vi "UHR-Fleezers Control (host) - 11.1.vi"() -> ()   [LabVIEW 2012] (continued)
        n1599 = feedback #34() -> (w2754:u32)  [unwired: 1 out]
        n1600 = case shown="True" w2761 {
          tunnel: [w2773 1] -> w2762
          tunnel: w2766 -> [w2775 _]
          tunnel: [w2774 w2793] -> w2763
          tunnel: w2764 -> [w2774 _]
          tunnel: w2760 -> [_ w2813]
          tunnel: w2753 -> [_ w2811]
          tunnel: w2755 -> [_ w2814]
          tunnel: [w2772 w2792] -> w2752
          tunnel: w2754 -> [w2772 _]
          tunnel: [w2771 w2790] -> w2749
          tunnel: w2750 -> [w2771 _]
          tunnel: [w2770 w2789] -> w2746
          tunnel: w2747 -> [w2770 _]
          tunnel: "Start Saving" -> [_ w2787]
          tunnel: w2742 -> [_ w2786]
          tunnel: [w2769 w2777] -> w2735
          tunnel: w2739 -> [w2769 _]
          tunnel: [w2768 w2776] -> w2736
          tunnel: w2737 -> [w2768 _]
          frame False {
            n1601 = Increment(x=w2775) -> (x+1=w2773:i32)
          }
          frame True {
            w2783 = FALSE ("Start Saving")
            w2788 = 9.0  # File Version
            w2796 = FALSE ("prepend array or string size? (T)")
            w2794 = T36."big-endian, network order" ("byte order (0:big-endian, network order)")
            n1602 = local read "BD 1 Frequency 1 (MHz)"() -> (w2810:dbl)
            n1603 = local read "BD 2 Frequency 1 (MHz)"() -> (w2809:dbl)
            n1604 = local read "BD 1 Frequency 2 (MHz)"() -> (w2808:dbl)
            n1605 = local read "BD 2 Frequency 2 (MHz)"() -> (w2807:dbl)
            n1606 = local read "BD 1 Frequency 3 (MHz)"() -> (w2806:dbl)
            n1607 = local read "BD 2 Frequency 3 (MHz)"() -> (w2805:dbl)
            n1608 = Array Size(array=w2786) -> (size(s)=w2785:i32)
            n1609 = To Double Precision Float(number=w2785) -> (double precision float=w2784:dbl)
            n1610 = local write "Save Calibration"(w2783) -> ()
            n1611 = local write "Start Saving"(w2783) -> ()
            n1612 = Build Array("Save APD Data\nwith Trap Data", "Save Trap Pos. Data") -> (w2780:bool[])
            n1613 = Boolean Array To Number(Boolean array=w2780) -> (number=w2779:u32)
            n1614 = Build Array(w2810, w2809, w2808, w2807, w2806, w2805) -> (w2804:dbl[])
            n1615 = case shown="1, Default" w2814 {
              tunnel: w2813 -> [w2885 w2905 w2921 w2959]
              tunnel: w2784 -> [w2890 w2912 w2941 w2978]
              tunnel: w2811 -> [w2889 w2911 w2940 w2977]
              tunnel: [w2886 w2907 w2932 w2969] -> w2802
              tunnel: [w2877 "Cal sets to save" w2922 w2960] -> w2792
              tunnel: w2804 -> [w2887 w2908 w2934 w2971]
              tunnel: "Save APD Data\nwith Trap Data" -> [w2884 _ w2918 w2957]
              tunnel: [w2884 w2899 w2918 w2957] -> w2789
              tunnel: w2788 -> [w2880 w2900 w2916 w2955]
              tunnel: w2787 -> [w2879 _ _ _]
              tunnel: [w2870 w2899 w2915 w2945] -> w2776
              tunnel: "Save Trap Pos. Data" -> [w2870 _ w2915 w2945]
              tunnel: w2779 -> [w2869 _ w2914 w2944]
              frame 1, Default {
                # "timeseries"
                n1616 = case shown="True" "Profile" {
                  tunnel: [w2893 w2897] -> w2874
                  tunnel: [w2893 w2896] -> w2873
                  tunnel: [w2893 w2895] -> w2872
                  tunnel: [w2893 w2894] -> w2871
                  frame False {
                    w2893 = 0.0 ("f")
                  }
                  frame True {
                    n1617 = local read "Current Position"() -> (w2898:cluster{dbl, dbl, dbl})
                    n1618 = local read "Y change (mm)"() -> (w2894:dbl)
                    n1619 = Unbundle(w2898) -> (w2897:dbl, w2896:dbl, w2895:dbl)
                  }
                }
                n1620 = local read "Save ave N"() -> (w2892:dbl)
                n1621 = Multiply(x=w2892, y=w2885) -> (x*y=w2891:dbl)
                n1622 = To Double Precision Float(number=w2869) -> (double precision float=w2883:dbl)
                n1623 = Build Array(w2880, w2885, w2891, w2890, w2889, 0.0 ("f")) -> (w2888:dbl[])
                n1624 = Build Array(w2883, w2874, w2873, w2872, w2871) -> (w2881:dbl[])
                n1625 = Select(t=u32 4000000000, s=w2879, f="N sets to save") -> (s? t:f=w2877:u32)
                n1626 = Build Array (concatenate)(w2888, w2887, w2881) -> (w2886:dbl[])
              }
              frame 2 {
                w2902 = 0.0 ("f")
                w2899 = FALSE ("Save APD Data\nwith Trap Data")
                # "calibration"
                n1627 = Boolean To (0,1)(Boolean=w2899) -> (0, 1=w2904:i16)
                n1628 = To Double Precision Float(number=w2904) -> (double precision float=w2903:dbl)
                n1629 = Build Array(w2903, w2902, w2902, w2902, w2902) -> (w2901:dbl[])
                n1630 = Build Array(w2900, w2905, w2905, w2912, w2911, 1.0 ("t")) -> (w2909:dbl[])
                n1631 = Build Array (concatenate)(w2909, w2908, w2901) -> (w2907:dbl[])
                "Calibrating Trap..." <- TRUE ("Calibrating...")
              }
              frame 4 {
                w2919 = 0.0 ("f")
                # "scan dir (x/y = 0/1)"
                # "cycles/step"
                # "n scans (f/b)"
                # "steps"
                # "freq. range"
                # "AOD raster scan"
                n1632 = local read "Number of F/B Scans (AOD)"() -> (w2926:u16)
                n1633 = local read "Cycles/step (AOD)"() -> (w2928:u64)
                n1634 = local read "Scan Range (MHz)"() -> (w2931:dbl)
                n1635 = local read "Scan steps (AOD)"() -> (w2930:u64)
                n1636 = local read "Scan BD"() -> (w2938:bool)
                n1637 = local read "Save ave N"() -> (w2943:dbl)
                n1638 = Boolean To (0,1)(Boolean=w2938) -> (0, 1=w2937:i16)
                n1639 = To Double Precision Float(number=w2926) -> (double precision float=w2925:dbl)
                n1640 = To Double Precision Float(number=w2930) -> (double precision float=w2929:dbl)
                n1641 = To Double Precision Float(number=w2928) -> (double precision float=w2927:dbl)
                n1642 = To Double Precision Float(number=w2937) -> (double precision float=w2936:dbl)
                n1643 = Multiply(x=w2943, y=w2921) -> (x*y=w2942:dbl)
                n1644 = To Double Precision Float(number=w2914) -> (double precision float=w2920:dbl)
                n1645 = Build Array(w2920, w2919, w2919, w2919, w2919) -> (w2917:dbl[])
                n1646 = local read "N sets should be saved"() -> (w2923:dbl)
                n1647 = Build Array(w2936, w2931, w2929, w2927, w2925) -> (w2933:dbl[])
                n1648 = Build Array(w2916, w2921, w2942, w2941, w2940, 2.0 ("t")) -> (w2935:dbl[])
                n1649 = Round Toward +Infinity(x=w2923) -> (ceil(x): smallest int >= x=w2924:dbl)
                n1650 = Build Array (concatenate)(w2935, w2934, w2917, w2933) -> (w2932:dbl[])
                n1651 = To Unsigned Long Integer(number=w2924) -> (unsigned 32bit integer=w2922:u32)
              }
              frame 8 {
                w2952 = 0.0 ("f")
                # "MCL raster scan"
                n1652 = local read "Number of scans (MCL)"() -> (w2947:u64)
                n1653 = local read "Scan lines (y)"() -> (w2946:u64)
                n1654 = local read "2D or 1D Scan"() -> (w2949:bool)
                n1655 = local read "Scan Range (V)\n(of steps)"() -> (w2968:dbl)
                n1656 = local read "Fast Scan Dir"() -> (w2975:bool)
                n1657 = local read "Cycles/step (MCL)"() -> (w2965:u64)
                n1658 = local read "Scan steps (MCL)"() -> (w2967:u64)
                n1659 = Select(t=w2946, s=w2949, f=w2947) -> (s? t:f=w2948:u64)
                n1660 = Boolean To (0,1)(Boolean=w2949) -> (0, 1=w2951:i16)
                n1661 = local read "Save ave N"() -> (w2980:dbl)
                n1662 = local read "Initial X"() -> (w2954:dbl)
                n1663 = local read "Initial Y"() -> (w2953:dbl)
                n1664 = To Double Precision Float(number=w2951) -> (double precision float=w2950:dbl)
                n1665 = Boolean To (0,1)(Boolean=w2975) -> (0, 1=w2974:i16)
                n1666 = To Double Precision Float(number=w2948) -> (double precision float=w2963:dbl)
                n1667 = To Double Precision Float(number=w2967) -> (double precision float=w2966:dbl)
                n1668 = To Double Precision Float(number=w2965) -> (double precision float=w2964:dbl)
                n1669 = To Double Precision Float(number=w2974) -> (double precision float=w2973:dbl)
                n1670 = Multiply(x=w2980, y=w2959) -> (x*y=w2979:dbl)
                n1671 = To Double Precision Float(number=w2944) -> (double precision float=w2958:dbl)
                n1672 = local read "N sets should be saved (MCL)"() -> (w2961:dbl)
                n1673 = Build Array(w2958, w2950, w2952, w2952, w2952) -> (w2956:dbl[])
                n1674 = Build Array(w2973, w2968, w2966, w2964, w2963, w2954, w2953) -> (w2970:dbl[])
                n1675 = Build Array(w2955, w2959, w2979, w2978, w2977, 3.0 ("t")) -> (w2972:dbl[])
                n1676 = Round Toward +Infinity(x=w2961) -> (ceil(x): smallest int >= x=w2962:dbl)
                n1677 = Build Array (concatenate)(w2972, w2971, w2956, w2970) -> (w2969:dbl[])
                n1678 = To Unsigned Long Integer(number=w2962) -> (unsigned 32bit integer=w2960:u32)
              }
            }
            n1679 = local read "Index"() -> (w2819:dbl)
            n1680 = call "Create new save file.vi"("Insert"="", "Ext"=".dat", "Index In"=w2819) -> ("Path Out"=w2778:path, "Index Out"=w2791:dbl)
            n1681 = local write "Save file name"(w2778) -> ()
            n1682 = local write "Index"(w2791) -> ()
            n1683 = local write "Save index"(w2791) -> ()
            n1684 = Array Size(array=w2802) -> (size(s)=w2803:i32)
            n1685 = Open/Create/Replace File(file path (use dialog)=w2778, operation (0:open)=T35."create", access (0:read/write)=enum16{"read/write", "read-only", "write-only"}."write-only") -> (refnum out=w2816:refnum<file>)  [unwired: 1 in, 4 out]
            n1686 = local write "Saving..."(TRUE ("Saving...")) -> ()
            n1687 = To Double Precision Float(number=w2803) -> (double precision float=w2801:dbl)
            n1688 = String Length(string="Comment (data description)") -> (length=w2799:i32)
            n1689 = To Double Precision Float(number=w2799) -> (double precision float=w2798:dbl)
            n1690 = Deny Access(7:w2816) -> (3:w2815:refnum<file>)  [unwired: 1 in, 2 out]
            n1691 = Build Array (concatenate)(w2801, w2802, w2798) -> (w2800:dbl[])
            n1692 = case "If fluorescence data to be saved" shown="True" w2789 {
              tunnel: w2778 -> [_ w2868]
              tunnel: [refnum<k0> refnum w2848] -> w2790
              frame False {
              }
              frame True {
                w2847 = 0.0
                n1693 = local read "APD Integration Time (s)"() -> (w2853:dbl)
                n1694 = local read "N APD Samp/step"() -> (w2846:dbl)
                n1695 = Path To String(path=w2868) -> (string=w2867:string)
                n1696 = String Length(string=w2867) -> (length=w2866:i32)
                n1697 = Subtract(x=w2866, y=4) -> (x-y=w2864:i32)
                n1698 = String Subset(string=w2867, length (rest)=w2864) -> (substring=w2863:string)  [unwired: 1 out]
                n1699 = Build Array(w2853, w2846, w2847, w2847, w2847, w2847, w2847, w2847) -> (w2850:dbl[])
                n1700 = Concatenate Strings(w2863, "_fl.dat" ("string")) -> (w2861:string)
                n1701 = Array Size(array=w2850) -> (size(s)=w2852:i32)
                n1702 = String To Path(string=w2861) -> (path=w2857:path)
                n1703 = Open/Create/Replace File(file path (use dialog)=w2857, operation (0:open)=T35."create", access (0:read/write)=enum16{"read/write", "read-only", "write-only"}."write-only") -> (refnum out=w2858:refnum<file>)  [unwired: 1 in, 4 out]
                n1704 = Deny Access(7:w2858) -> (3:w2854:refnum<file>)  [unwired: 1 in, 2 out]
                n1705 = To Double Precision Float(number=w2852) -> (double precision float=w2851:dbl)
                n1706 = Build Array (concatenate)(w2851, w2850) -> (w2849:dbl[])
                n1707 = Write to Binary File(file (use dialog)=w2854, data=w2849, 5:FALSE ("prepend array or string size? (T)"), 9:T36."big-endian, network order" ("byte order (0:big-endian, network order)")) -> (refnum out=w2848:refnum<file>)  [unwired: 1 in, 3 out]
              }
            }
            n1708 = case shown="True" w2776 {
              tunnel: w2778 -> [_ w2830]
              tunnel: [refnum<k0> refnum w2829] -> w2777
              frame False {
              }
              frame True {
                w2825 = 0.0 ("element")
                n1709 = Path To String(path=w2830) -> (string=w2844:string)
                n1710 = Build Array(w2825, w2825, w2825, w2825, w2825, w2825, w2825, w2825) -> (w2826:dbl[])
                n1711 = String Length(string=w2844) -> (length=w2843:i32)
                n1712 = Subtract(x=w2843, y=4) -> (x-y=w2841:i32)
                n1713 = Array Size(array=w2826) -> (size(s)=w2828:i32)
                n1714 = String Subset(string=w2844, length (rest)=w2841) -> (substring=w2840:string)  [unwired: 1 out]
                n1715 = To Double Precision Float(number=w2828) -> (double precision float=w2827:dbl)
                n1716 = Concatenate Strings(w2840, "_pos.dat" ("string")) -> (w2838:string)
                n1717 = Build Array (concatenate)(w2827, w2826) -> (w2824:dbl[])
                n1718 = String To Path(string=w2838) -> (path=w2834:path)
                n1719 = Open/Create/Replace File(file path (use dialog)=w2834, operation (0:open)=T35."create", access (0:read/write)=enum16{"read/write", "read-only", "write-only"}."write-only") -> (refnum out=w2835:refnum<file>)  [unwired: 1 in, 4 out]
                n1720 = Deny Access(7:w2835) -> (3:w2831:refnum<file>)  [unwired: 1 in, 2 out]
                n1721 = Write to Binary File(file (use dialog)=w2831, data=w2824, 5:FALSE ("prepend array or string size? (T)"), 9:T36."big-endian, network order" ("byte order (0:big-endian, network order)")) -> (refnum out=w2829:refnum<file>)  [unwired: 1 in, 3 out]
              }
            }
            n1722 = Write to Binary File(file (use dialog)=w2815, data=w2800, 5:w2796, 9:w2794) -> (refnum out=w2797:refnum<file>)  [unwired: 1 in, 3 out]
            n1723 = Write to Binary File(file (use dialog)=w2797, data="Comment (data description)", 5:w2796, 9:w2794) -> (refnum out=w2793:refnum<file>)  [unwired: 1 in, 3 out]
          }
        }
        n1724 = feedback-in #28(w2736) -> ()
        n1725 = feedback-in #29(w2763) -> ()
        n1726 = feedback-in #30(w2735) -> ()
        n1727 = feedback-in #31(w2746) -> ()
        n1728 = feedback-in #32(w2749) -> ()
        n1729 = feedback-in #33(w2762) -> ()
        n1730 = feedback-in #34(w2752) -> ()
      }
      frame #1 {
        n1731 = local read "Saving..."() -> (w2994:bool)
        n1732 = case shown="True" w2994 {
          tunnel: w2998 -> [_ w3009]
          tunnel: w2997 -> [_ w3023]
          tunnel: w2996 -> [_ w3019]
          tunnel: w2995 -> [_ w3018]
          tunnel: w2993 -> [_ w3017]
          tunnel: w2992 -> [_ w3012]
          tunnel: w2991 -> [_ w3011]
          tunnel: w2990 -> [_ w3010]
          tunnel: w2989 -> [_ w3008]
          tunnel: w2988 -> [_ w3006]
          tunnel: w2987 -> [_ w3005]
          tunnel: w2986 -> [_ w3004]
          tunnel: w2985 -> [_ w3003]
          tunnel: w2984 -> [_ w3002]
          tunnel: w2983 -> [_ w3001]
          tunnel: w2982 -> [_ w3000]
          tunnel: w2981 -> [_ w2999]
          frame False {
          }
          frame True {
            n1733 = Multiply(x=w3009, y=w3008) -> (x*y=→"Time (s)":dbl)
            n1734 = Less Or Equal?(x=w3009, y=w3017) -> (x <= y?=w3021:bool)
            n1735 = Or(x="Stop Saving", y="Abort save 2") -> (x .or. y?=w3013:bool)
            n1736 = Not(x=w3013) -> (.not. x?=w3022:bool)
            n1737 = And(x=w3021, y=w3022) -> (x .and. y?=w3020:bool)
            n1738 = case shown="True" w3020 {
              tunnel: w3023 -> [w3030 w3105]
              tunnel: [0.0 w3108] -> w3016
              tunnel: w3009 -> [_ w3106]
              tunnel: w3017 -> [_ w3107]
              tunnel: w3019 -> [_ w3102]
              tunnel: w3018 -> [_ _]
              tunnel: w3012 -> [w3028 w3095]
              tunnel: w3011 -> [w3027 w3096]
              tunnel: w3010 -> [_ w3094]
              tunnel: w3006 -> [_ w3093]
              tunnel: w3005 -> [_ w3037]
              tunnel: w3004 -> [_ w3086]
              tunnel: w3003 -> [_ w3064]
              tunnel: w3002 -> [w3024 w3046]
              tunnel: w3001 -> [w3025 w3045]
              tunnel: w3000 -> [_ w3042]
              tunnel: w2999 -> [_ w3040]
              frame False {
                w3026 = FALSE
                n1739 = Close File(refnum=w3030) -> ()  [unwired: 1 in, 2 out]
                n1740 = case shown="True" w3027 {
                  tunnel: w3028 -> [_ w3032]
                  frame False {
                  }
                  frame True {
                    n1741 = Close File(refnum=w3032) -> ()  [unwired: 1 in, 2 out]
                  }
                }
                n1742 = case shown="True" w3024 {
                  tunnel: w3025 -> [_ w3031]
                  frame False {
                  }
                  frame True {
                    n1743 = Close File(refnum=w3031) -> ()  [unwired: 1 in, 2 out]
                  }
                }
                n1744 = local write "Raster Scanning..."(w3026) -> ()
                n1745 = local write "Calibrating Trap..."(w3026) -> ()
                n1746 = call <vilib>:"Beep.vi"() -> ()  [unwired: 3 in, 9 out]
                n1747 = local write "Stop Saving"(w3026) -> ()
                "Saving..." <- w3026
              }
              frame True {
                n1748 = local read "Calibrating Trap..."() -> (w3097:bool)
                n1749 = case "Write fl. data" shown="True" w3096 {
                  tunnel: w3095 -> [_ w3131]
                  tunnel: w3094 -> [_ w3130]
                  frame False {
                  }
                  frame True {
                    n1750 = Write to Binary File(file (use dialog)=w3131, data=w3130, 5:FALSE ("prepend array or string size? (T)"), 9:T36."big-endian, network order" ("byte order (0:big-endian, network order)")) -> ()  [unwired: 1 in, 4 out]
                  }
                }
                n1751 = Greater?(x="Save ave N", y=1.0) -> (0:w3100:bool)
                n1752 = Not(x=w3097) -> (.not. x?=w3099:bool)
                n1753 = And(x=w3099, y=w3100) -> (x .and. y?=w3043:bool)
                n1754 = case shown="True" w3043 {
                  tunnel: w3042 -> [w3111 w3122]
                  tunnel: [w3111 w3114] -> w3041
                  tunnel: "Save ave N" -> [_ w3115]
                  frame False {
                  }
                  frame True {
                    w3112 = 2 ("dimension size")
                    n1755 = Array Size(array=w3122) -> (size(s)=w3116:i32)
                    n1756 = Divide(x=w3116, y=w3112) -> (x/y=w3120:dbl)
                    n1757 = Reshape Array(w3122, w3120, w3112) -> (w3121:u64[][])
                    n1758 = Transpose 2D Array(2D array=w3121) -> (transposed array=w3119:u64[][])
                    n1759 = for {
                      tunnel: w3119 -> [w3124] mode=indexing
                      tunnel: [w3123] -> w3113 mode=indexing
                      tunnel: w3115 -> [w3125]
                      workers-P: _ -> [_]
                      n1760 = call "downsample 1D array - U64.vi"("Ave N"=w3125, "Array In"=w3124) -> ("Array Out"=w3123:u64[])  [unwired: 1 in]
                    }
                    n1761 = Transpose 2D Array(2D array=w3113) -> (transposed array=w3118:u64[][])
                    n1762 = Divide(x=w3116, y=w3115) -> (x/y=w3117:dbl)
                    n1763 = Reshape Array(w3118, w3117) -> (w3114:u64[])
                  }
                }
                n1764 = case shown="True" w3043 {
                  tunnel: w3102 -> [w3134 w3146]
                  tunnel: [w3134 w3138] -> w3098
                  tunnel: "Save ave N" -> [_ w3139]
                  tunnel: w3093 -> [_ w3137]
                  frame False {
                  }
                  frame True {
                    n1765 = Array Size(array=w3146) -> (size(s)=w3140:i32)
                    n1766 = Array Size(array=w3137) -> (size(s)=w3136:i32)
                    n1767 = Divide(x=w3140, y=w3136) -> (x/y=w3144:dbl)
                    n1768 = Reshape Array(w3146, w3144, w3136) -> (w3145:i16[][])
                    n1769 = Transpose 2D Array(2D array=w3145) -> (transposed array=w3143:i16[][])
                    n1770 = for {
                      tunnel: w3143 -> [w3149] mode=indexing
                      tunnel: [w3148] -> w3135 mode=indexing
                      tunnel: w3139 -> [w3147]
                      workers-P: _ -> [_]
                      n1771 = call "downsample 1D array - I16.vi"("Ave N"=w3147, "Array In"=w3149) -> ("Array Out"=w3148:i16[])  [unwired: 1 out]
                    }
                    n1772 = Transpose 2D Array(2D array=w3135) -> (transposed array=w3142:i16[][])
                    n1773 = Divide(x=w3140, y=w3139) -> (x/y=w3141:dbl)
                    n1774 = Reshape Array(w3142, w3141) -> (w3138:i16[])
                  }
                }
                n1775 = Index Array(array=w3064, index=1) -> (element=w3067:waveform(dbl))
                n1776 = Index Array(array=w3064, index=0) -> (element=w3069:waveform(dbl))
                n1777 = Unbundle By Name(w3067) -> ("Y"=w3071:dbl[])
                n1778 = Unbundle By Name(w3069) -> ("Y"=w3079:dbl[])
                n1779 = case "Write trap pos. data" shown="True" w3046 {
                  tunnel: w3045 -> [_ w3127]
                  tunnel: w3041 -> [_ w3126]
                  frame False {
                  }
                  frame True {
                    n1780 = Write to Binary File(file (use dialog)=w3127, data=w3126, 5:FALSE ("prepend array or string size? (T)"), 9:T36."big-endian, network order" ("byte order (0:big-endian, network order)")) -> ()  [unwired: 1 in, 4 out]
                  }
                }
                n1781 = Write to Binary File(file (use dialog)=w3105, data=w3098, 5:FALSE ("prepend array or string size? (T)"), 9:T36."big-endian, network order" ("byte order (0:big-endian, network order)")) -> ()  [unwired: 1 in, 4 out]
                n1782 = feedback #35(w3071) -> (w3073:dbl[])
                n1783 = Build Array (concatenate)(w3073, w3071) -> (w3072:dbl[])
                n1784 = Select(t=w3071, s=w3037, f=w3072) -> (s? t:f=w3057:dbl[])
                n1785 = feedback-in #35(w3057) -> ()
                n1786 = feedback #36(w3079) -> (w3092:dbl[])
                n1787 = Build Array (concatenate)(w3092, w3079) -> (w3091:dbl[])
                n1788 = Select(t=w3079, s=w3037, f=w3091) -> (s? t:f=w3066:dbl[])
                n1789 = feedback-in #36(w3066) -> ()
                n1790 = Divide(x=w3106, y=w3107) -> (x/y=w3109:dbl)
                n1791 = Multiply(x=w3109, y=100.0) -> (x*y=w3108:dbl)
                n1792 = Build Array(w3066, w3057) -> (→"Saved APD":dbl[][])
                n1793 = Array Size(array=w3066) -> (size(s)=w3084:i32)
                n1794 = Unbundle By Name(w3086) -> ("Y"=w3090:dbl[])
                n1795 = Subtract(x=w3084, y="N pts to average") -> (x-y=w3060:i32)
                n1796 = Multiply(x="N pts to average", y=u16 2) -> (x*y=w3061:u16)
                n1797 = Subtract(x=w3084, y=w3061) -> (x-y=w3059:i32)
                n1798 = feedback #37(w3090) -> (w3089:dbl[])
                n1799 = Build Array (concatenate)(w3089, w3090) -> (w3088:dbl[])
                n1800 = Select(t=w3090, s=w3037, f=w3088) -> (s? t:f=w3087:dbl[])
                "Trap Delta Graph" <- w3087
                n1801 = feedback-in #37(w3087) -> ()
                n1802 = Array Subset(array=w3066, index=w3060, length="N pts to average") -> (w3083:dbl[])
                n1803 = Array Subset(array=w3066, index=w3059, length="N pts to average") -> (w3082:dbl[])
                n1804 = Array Subset(array=w3057, index=w3060, length="N pts to average") -> (w3063:dbl[])
                n1805 = Array Subset(array=w3057, index=w3059, length="N pts to average") -> (w3062:dbl[])
                n1806 = Index Array(array=w3040, index=0) -> (element=w3038:waveform(dbl))
                n1807 = call-poly <vilib>:"Mean.vi"("X"=w3083) -> ("mean"=w3081:dbl)  [unwired: 1 out]
                n1808 = call-poly <vilib>:"Mean.vi"("X"=w3063) -> ("mean"=w3056:dbl)  [unwired: 1 out]
                n1809 = call-poly <vilib>:"Mean.vi"("X"=w3082) -> ("mean"=w3080:dbl)  [unwired: 1 out]
                n1810 = call-poly <vilib>:"Mean.vi"("X"=w3062) -> ("mean"=w3055:dbl)  [unwired: 1 out]
                n1811 = Unbundle By Name(w3038) -> ("Y"=w3035:dbl[])
                n1812 = Subtract(x=w3056, y=w3055) -> (x-y=w3047:dbl)
                "Delta Fl. 2" <- w3047
                n1813 = Subtract(x=w3081, y=w3080) -> (x-y=w3078:dbl)
                "Delta Fl. 1" <- w3078
                n1814 = Initialize Array(w3078, 1 ("dimension size")) -> (w3075:dbl[])
                n1815 = Initialize Array(w3047, 1 ("dimension size")) -> (w3052:dbl[])
                n1816 = feedback #38(w3075) -> (w3076:dbl[])
                n1817 = Build Array (concatenate)(w3076, w3075) -> (w3074:dbl[])
                n1818 = feedback #39(w3052) -> (w3053:dbl[])
                n1819 = Build Array (concatenate)(w3053, w3052) -> (w3051:dbl[])
                n1820 = feedback #40(w3035) -> (w3034:dbl[])
                n1821 = Build Array (concatenate)(w3034, w3035) -> (w3036:dbl[])
                n1822 = Select(t=w3035, s=w3037, f=w3036) -> (s? t:f=w3033:dbl[])
                "Saved trap pos" <- w3033
                n1823 = feedback-in #40(w3033) -> ()
                n1824 = Select(t=w3075, s=w3037, f=w3074) -> (s? t:f=w3050:dbl[])
                n1825 = feedback-in #38(w3050) -> ()
                n1826 = Select(t=w3052, s=w3037, f=w3051) -> (s? t:f=w3049:dbl[])
                n1827 = feedback-in #39(w3049) -> ()
                n1828 = Build Array(w3050, w3049) -> (→"Save APD Deriv":dbl[][])
              }
            }
            "Progress" <- w3016
            "Progress 2" <- w3016
          }
        }
      }
    }
    n1829 = Bundle By Name(cluster=w1676, "Green FB Ch 0"=w1675, "Green FB Ch 1"=w1674) -> (w1654:T44)
    "Green FB Signals (V)" <- w1654
    n1830 = Unbundle By Name(w1654) -> ("Green FB Ch 2"=→"Green FB Plot":dbl)
    n1831 = local read "wait to reset values"() -> (w1745:bool)
    n1832 = Not(x=w1743) -> (.not. x?=w1746:bool)
    n1833 = And(x=w1746, y=w1745) -> (x .and. y?=w1747:bool)
    n1834 = case "Part of MCL raster scanning: returns to initial positions after scan done" shown="True" w1747 {
      tunnel: w1460 -> [w2556 w2563]
      tunnel: [w2556 w2562] -> w1749
      tunnel: w1459 -> [w2555 w2561]
      tunnel: [w2555 w2560] -> w1744
      frame False {
      }
      frame True {
        w2571 = 10.0 ("y")
        w2570 = 32767.0 ("y")
        # "to return scan values\nafter a synchronous \nAOM scan"
        n1835 = local read "AO2"() -> (w2564:dbl)
        n1836 = local read "AO1"() -> (w2565:dbl)
        n1837 = local write "wait to reset values"(FALSE ("wait to reset values")) -> ()
        n1838 = Multiply(x=w2565, y=w2570) -> (x*y=w2567:dbl)
        n1839 = Multiply(x=w2564, y=w2570) -> (x*y=w2569:dbl)
        n1840 = Divide(x=w2567, y=w2571) -> (x/y=w2566:dbl)
        n1841 = Divide(x=w2569, y=w2571) -> (x/y=w2568:dbl)
        n1842 = To Word Integer(number=w2566) -> (16bit integer=w2572:i16)
        n1843 = To Word Integer(number=w2568) -> (16bit integer=w2573:i16)
        n1844 = local read "Total Counts (ticks)"() -> (w2557:u32)
        n1845 = xnode "Read/Write Control"("FPGA VI Reference In"=w2563, "error in"=w2561, "AO1"=w2572, "AO2"=w2573, "MCL count"=w2557) -> ("FPGA VI Reference Out"=w2562:T19, "error out"=w2560:errorcluster)
        n1846 = local read "Scan Range (V)\n(of steps)"() -> (w2558:dbl)
        n1847 = property on="Scan Range (V)\n(of steps)" class="DigNum (strict)"("Val(Sgnl)"=w2558) -> ()  [unwired: 2 in, 2 out]
      }
    }
    n1848 = node-c288() -> ()  [unwired: 2 out]
  }
  n1849 = timed-loop "Control parameters (event loop)" {
    tunnel: w6 -> [w3158]
    shift-right: [w3157] -> _
    shift-left: errorcluster {"status"=FALSE, "code"=0, "source"=""} ("error out") -> [w3156]
    tunnel: [w3155] -> _
    timing: w97 -> [_]
    timing-out: [_] -> w96
    tunnel: w69 -> [w3154]
    tunnel: w10 -> [w3153]
    tunnel: w9 -> [w3152]
    tunnel: w8 -> [w3151]
    tunnel: w7 -> [w3150]
    stop <- w3155 stop-if-true
    n1850 = node-c288() -> ()  [unwired: 2 out]
    n1851 = event shown="[75] \"Trap pos\": Value Change" {
      selector: _ -> [_ _ _ _ _ _ _ _ _ _ _ _ _ _ _ _ _ _ _ _ _ _ _ _ _ _ _ _ _ _ _ _ _ _ _ _ _ _ _ _ _ _ _ _ _ _ _ _ _ _ _ _ _ _ _ _ _ _ _ _ _ _ _ _ _ _ _ _ _ _ _ _ _ _ _ _]
      dyn-events: _ -> [_ _ _ _ _ _ _ _ _ _ _ _ _ _ _ _ _ _ _ _ _ _ _ _ _ _ _ _ _ _ _ _ _ _ _ _ _ _ _ _ _ _ _ _ _ _ _ _ _ _ _ _ _ _ _ _ _ _ _ _ _ _ _ _ _ _ _ _ _ _ _ _ _ _ _ _]
      timeout: _ -> [_ _ _ _ _ _ _ _ _ _ _ _ _ _ _ _ _ _ _ _ _ _ _ _ _ _ _ _ _ _ _ _ _ _ _ _ _ _ _ _ _ _ _ _ _ _ _ _ _ _ _ _ _ _ _ _ _ _ _ _ _ _ _ _ _ _ _ _ _ _ _ _ _ _ _ _]
      tunnel: w3158 -> [w3196 _ _ _ w3234 _ w3256 _ _ _ _ w3322 _ _ w3365 w3371 w3376 w3382 w3418 w3436 w3443 _ w3455 w3459 w3470 w3481 w3492 w3503 w3514 w3525 w3552 w3646 w3653 w3691 _ w3726 w3730 w3741 w3745 w3749 _ w3757 _ _ _ _ _ _ _ _ _ _ _ _ _ _ _ _ _ w4135 _ w4152 _ w4159 w4177 _ w4184 w4192 w4207 w4218 w4224 _ w4233 _ w4252 _]
      tunnel: [w3195 _ _ _ w3224 _ w3255 _ _ w3287 _ w3301 _ _ w3364 w3367 w3373 w3379 w3417 w3434 w3442 _ w3453 _ w3464 w3475 w3486 w3497 w3508 w3519 w3550 w3644 w3651 w3689 _ w3724 w3728 w3731 w3743 w3747 _ w3755 _ _ _ _ _ _ _ _ _ _ _ _ _ _ _ _ _ w4133 _ _ _ _ w4174 _ _ _ _ _ _ _ _ _ _ _] -> w3157
      tunnel: w3156 -> [w3194 _ _ _ w3233 _ w3254 _ _ w3287 _ w3321 _ _ w3363 w3366 w3372 w3378 w3416 w3435 w3441 _ w3454 w3458 w3469 w3480 w3491 w3502 w3513 w3524 w3551 w3645 w3652 w3690 _ w3725 w3729 w3740 w3744 w3748 _ w3756 _ _ _ _ _ _ _ _ _ _ _ _ _ _ _ _ _ w4134 _ w4151 _ w4158 w4176 _ w4183 w4191 w4206 w4217 w4223 _ w4232 _ w4251 _]
      tunnel: [_ _ _ _ _ _ _ _ _ w3286 _ _ _ _ _ _ _ _ _ _ _ _ _ _ _ _ _ _ _ _ _ _ _ _ _ _ _ _ _ _ _ _ _ _ _ _ _ _ _ _ _ _ _ _ _ _ _ _ _ _ _ _ _ _ _ _ _ _ _ _ _ _ _ _ _ _] -> w3155
      tunnel: [_ _ _ _ _ _ _ "Round T1 X" _ _ _ _ _ _ _ _ _ _ _ _ _ _ _ _ _ _ _ _ _ _ _ _ _ _ _ _ _ _ _ _ _ _ _ _ _ _ _ _ _ _ _ _ _ _ _ _ _ _ _ _ _ _ _ _ _ _ _ _ _ _ _ _ _ _ _ _] -> _
      tunnel: [_ _ _ "Adjust Scale\nto Mean" _ _ _ _ _ _ _ _ _ _ _ _ _ _ _ _ _ _ "Test ttrig" _ _ _ _ _ _ _ _ _ _ _ _ _ _ _ _ _ _ _ _ _ _ _ _ _ _ "Flush Sample" "Flush Pump 3" "Flush Pump 1" "Clear Volume" _ _ _ _ _ _ _ _ _ _ _ _ _ _ _ _ _ _ _ _ _ _ _] -> _
      tunnel: [_ _ _ _ _ _ _ _ "Round T2 X" _ "Delayed Interlace Start" _ _ _ _ _ _ _ _ _ _ _ _ _ _ _ _ _ _ _ _ _ _ _ _ _ _ _ _ _ _ _ _ _ _ _ _ _ _ _ _ _ _ _ _ _ _ _ _ _ _ _ _ _ _ _ _ _ _ _ _ _ _ _ _ _] -> _
      tunnel: w3154 -> [_ _ _ _ _ _ _ _ _ _ _ _ _ _ _ _ _ _ _ _ _ _ _ _ _ _ _ _ _ _ _ _ _ _ _ _ _ _ _ _ _ _ _ _ _ w3914 w3921 w3928 w3933 w3942 _ _ w4048 _ _ _ _ _ _ _ _ _ _ _ _ _ _ _ _ _ _ _ _ _ _ _]
      tunnel: w3153 -> [_ _ _ _ _ _ _ _ _ _ _ _ _ _ _ _ _ _ _ _ _ _ _ _ _ _ _ _ _ _ _ _ _ _ _ _ _ _ _ _ _ _ _ w3831 _ _ _ _ _ _ w3986 _ _ w4054 _ w4063 _ w4077 _ _ _ _ _ _ _ _ _ _ _ _ _ _ _ _ _ _]
      tunnel: w3152 -> [_ _ _ _ _ _ _ _ _ _ _ _ _ _ _ _ _ _ _ _ _ _ _ _ _ _ _ _ _ _ _ _ _ _ _ _ _ _ _ _ _ _ _ _ _ _ _ _ _ _ _ _ _ _ _ _ _ _ _ _ _ _ _ _ _ _ _ _ _ _ _ _ _ _ _ _]
      tunnel: w3151 -> [_ _ _ _ _ _ _ _ _ _ _ _ _ _ _ _ _ _ _ _ _ _ _ _ _ _ _ _ _ _ _ _ _ _ _ _ _ _ _ _ _ _ w3768 _ _ _ _ _ _ _ _ w4016 _ _ w4059 _ w4070 _ w4102 _ _ _ _ _ _ _ _ _ _ _ _ _ _ _ _ _]
      tunnel: w3150 -> [_ _ _ _ _ _ _ _ _ _ _ _ _ _ _ _ _ _ _ _ _ _ _ _ _ _ _ _ _ _ _ _ _ _ _ _ _ _ _ _ _ _ _ _ _ _ _ _ _ _ _ _ _ _ _ _ _ _ _ _ _ _ _ _ _ _ _ _ _ _ _ _ _ _ _ _]
      event "AI Count (ticks)", "Sets to FIFO (Traps)", "Save ave N", "FPGA Ave.", "# Samples/channel", "N sets to save": Value Change {
        # "So that if 'Save ave N' is updated, the AOD scanning code updates too."
        n1852 = event-data() -> ()  [unwired: 6 out]
        n1853 = local read "AI Count (ticks)"() -> (w3176:u32)
        n1854 = Boolean To (0,1)(Boolean="Sets to FIFO (Traps)") -> (0, 1=w3186:cluster{"Set 1":i16, "Set 2":i16, "Set 3":i16})
        n1855 = xnode "Read/Write Control"("FPGA VI Reference In"=w3196, "error in"=w3194, "ai count"=w3176, "AI1 Sets to FIFO"="Sets to FIFO (Traps)", "N of AI1 Int Acq Sets"="N Acq Sets (Traps + Fl.)") -> ("error out"=w3195:errorcluster)  [unwired: 1 out]
        n1856 = Cluster To Array(cluster=w3186) -> (array=w3185:i16[])
        n1857 = To Unsigned Long Integer(number=w3185) -> (unsigned 32bit integer=w3165:u32[])
        n1858 = local read "Scan steps (AOD)"() -> (w3187:u64)
        n1859 = Multiply(x=w3176, y="N Acq Sets (Traps + Fl.)") -> (x*y=w3174:u32)
        n1860 = Divide(x=40000000.0, y=w3176) -> (x/y=w3168:dbl)
        "AI rate (Hz)" <- w3168
        "Ave. Rate (Hz)" <- w3168
        n1861 = Add Array Elements(numeric array=w3165) -> (sum=w3177:u32)
        "Trap Sets" <- w3177
        n1862 = Reciprocal(x=w3168) -> (1/x=→"Ave. Period (s)":dbl)
        n1863 = property on="Scan steps (AOD)" class="DigNum (strict)"("Val(Sgnl)"=w3187) -> ()  [unwired: 2 in, 2 out]
        n1864 = Divide(x=w3168, y="N Acq Sets (Traps + Fl.)") -> (x/y=w3191:dbl)
        "Data Rate (Hz)" <- w3191
        n1865 = Reciprocal(x=w3191) -> (1/x=→"Data Period (s)":dbl)
        n1866 = local read "Save ave N"() -> (w3190:dbl)
        n1867 = Divide(x=w3191, y=w3190) -> (x/y=w3189:dbl)
        "Save Data Rate (Hz)" <- w3189
        n1868 = Reciprocal(x=w3189) -> (1/x=→"Save Data Period (s)":dbl)
        n1869 = Multiply(x=w3174, y="# Samples/trap") -> (x*y=w3172:u32)
        "Counts/DMA" <- w3172
        n1870 = property on="Trap Disp. Downsample" class="DigNum (strict)"("Maximum"="# Samples/trap") -> ()  [unwired: 2 in, 2 out]
        n1871 = Multiply(x=w3177, y="# Samples/trap") -> (x*y=w3166:u32)
        "# Samples/channel" <- w3166
        n1872 = Multiply(x=w3166, y=u32 8) -> (x*y=→"Trap AI Elements/DMA read":u32)
        n1873 = local read "APD Int. Count"() -> (w3173:u32)
        n1874 = Multiply(x=w3166, y=u32 3) -> (x*y=→"Trap Pos Elements/DMA read":u32)
        n1875 = Divide(x=w3172, y=w3173) -> (x/y=w3163:dbl)
        "APD Samples/FIFO Acq." <- w3163
        n1876 = Divide(x=w3172, y=40000000.0) -> (x/y=w3170:dbl)
        "DMA Update Period (s)" <- w3170
        n1877 = Multiply(x=2.0, y=w3163) -> (x*y=→"APD Elements/DMA read":dbl)
        n1878 = property on="APD Disp. Downsample" class="DigNum (strict)"("Maximum"=w3163) -> ()  [unwired: 2 in, 2 out]
        n1879 = local read "N sets to save"() -> (w3183:u32)
        n1880 = Multiply(x=w3170, y=w3183) -> (x*y=→"Total Time (s)":dbl)
        "FPGA Averaging" <- FALSE ("FPGA Averaging")
      }
      event "Remove Offset": Value Change {
        n1881 = event-data() -> ()  [unwired: 7 out]
        n1882 = local write "Remove Offset"(FALSE ("Remove Offset")) -> ()
        n1883 = local read "Bead Mean (nm)"() -> (w3198:dbl)
        n1884 = local read "Offset (nm)"() -> (w3199:dbl)
        n1885 = Add(x=w3198, y=w3199) -> (x+y=w3197:dbl)
        n1886 = local write "Offset (nm)"(w3197) -> ()
        n1887 = disable-structure shown="Disabled" {
          frame Disabled {
            n1888 = local read "Bead Mean (nm)"() -> (w3204:dbl)
            n1889 = Add(y=w3204) -> (x=w3203:dbl, x+y=w3202:dbl)
            n1890 = Subtract(x=w3204, y=w3203) -> (x-y=w3201:dbl)
            n1891 = property on="Bead Separation" class="WFChart (strict)"("YScale.Minimum"=w3201) -> ()  [unwired: 2 in, 2 out]
            n1892 = property on="Bead Separation" class="WFChart (strict)"("YScale.Maximum"=w3202) -> ()  [unwired: 2 in, 2 out]
          }
          frame Enabled {
          }
        }
      }
      event "Detector Type": Value Change {
        n1893 = event-data() -> ()  [unwired: 7 out]
        n1894 = local read "AI labels"() -> (w3205:string[])
        n1895 = property on="High Res. Display" class="Ring (strict)"("Strings []"=w3205) -> ()  [unwired: 2 in, 2 out]
        n1896 = Build Array (concatenate)(w3205, "none") -> (w3206:string[])
        n1897 = property on="FFT 1 Choice 1" class="Ring (strict)"("Strings []"=w3206) -> ()  [unwired: 2 in, 2 out]
        n1898 = property on="FFT 1 Choice 2" class="Ring (strict)"("Strings []"=w3206) -> ()  [unwired: 2 in, 2 out]
        n1899 = property on="FFT 2 Choice 1" class="Ring (strict)"("Strings []"=w3206) -> ()  [unwired: 2 in, 2 out]
        n1900 = property on="FFT 2 Choice 2" class="Ring (strict)"("Strings []"=w3206) -> ()  [unwired: 2 in, 2 out]
        n1901 = Bundle("APD 1", "APD 2") -> (w3209:cluster{string, string})  [unwired: 1 out]
        n1902 = Cluster To Array(cluster=w3209) -> (array=w3207:string[])
        n1903 = Build Array (concatenate)(w3207, w3206) -> (w3211:string[])
        n1904 = Array Size(array=w3211) -> (size(s)=w3212:i32)
        n1905 = property on="Signals to Plot" class="LstBox (strict)"("Item Names"=w3211) -> ()  [unwired: 2 in, 2 out]
        n1906 = property on="Signals to Plot" class="LstBox (strict)"("Number of Rows"=w3212) -> ()  [unwired: 2 in, 2 out]
        n1907 = property on="All Signals" class="WFChart (strict)"("LegNumRows"=w3212) -> ()  [unwired: 2 in, 2 out]
      }
      event "Adjust Scale\nto Mean": Value Change {
        n1908 = event-data() -> ()  [unwired: 7 out]
        n1909 = local read "APD 1 Rate (Hz)"() -> (w3221:dbl)
        n1910 = Multiply(x=1000.0, y="Above (kHz)") -> (x*y=w3219:dbl)
        n1911 = Multiply(x=1000.0, y="Below (kHz)") -> (x*y=w3217:dbl)
        n1912 = Add(x=w3219, y=w3221) -> (x+y=w3214:dbl)
        n1913 = Subtract(x=w3221, y=w3217) -> (x-y=w3215:dbl)
        n1914 = property on="APD Chart" class="WFChart (strict)"("YScale.Minimum"=w3215) -> ()  [unwired: 2 in, 2 out]
        n1915 = property on="APD Chart" class="WFChart (strict)"("YScale.Maximum"=w3214) -> ()  [unwired: 2 in, 2 out]
      }
      event "Phase adj. (AI1)", "+ phase (AI1)", "- phase (AI1)": Value Change {
        n1916 = event-data() -> ()  [unwired: 7 out]
        n1917 = Negate(x="Phase adj. (AI1)") -> (-x=w3231:i16)
        n1918 = Select(t=w3231, s="- phase (AI1)", f="Phase adj. (AI1)") -> (s? t:f=w3230:i16)
        n1919 = xnode "Read/Write Control"("FPGA VI Reference In"=w3234, "error in"=w3233, "Phase count adjustment"=w3230) -> ("FPGA VI Reference Out"=w3229:T19, "error out"=w3228:errorcluster)
        n1920 = Or(x="- phase (AI1)", y="+ phase (AI1)") -> (x .or. y?=w3225:bool)
        n1921 = xnode "Read/Write Control"("FPGA VI Reference In"=w3229, "error in"=w3228, "+ phase"=w3225) -> ("error out"=w3224:errorcluster)  [unwired: 1 out]
      }
      event "Signals to Plot": Double Click {
        w3237 = u32 9868950 ("Color Box")
        n1922 = event-data() -> ("Row"=w3239:i32)  [unwired: 9 out]
        n1923 = property on="All Signals" class="WFChart (strict)"("Active Plot"=w3239) -> (error out=w3250:errorcluster)  [unwired: 2 in, 1 out]
        n1924 = property on="All Signals" class="WFChart (strict)" props=["Plot", "Visible?", "Plot", "Plot Color"](error in=w3250) -> (error out=w3249:errorcluster, "Plot.Visible?"=w3248:bool)  [unwired: 1 in, 2 out]
        n1925 = Select(t=FALSE ("Plot.Visible"), s=w3248, f=TRUE ("Plot.Visible")) -> (s? t:f=w3243:bool)
        n1926 = property on="All Signals" class="WFChart (strict)"(error in=w3249, "Plot.Visible?"=w3243) -> (error out=w3245:errorcluster)  [unwired: 1 in, 1 out]
        n1927 = property on="All Signals" class="WFChart (strict)"(error in=w3245) -> (error out=w3240:errorcluster, "Plot.Plot Color"=w3244:u32)  [unwired: 1 in, 1 out]
        n1928 = property on="Signals to Plot" class="LstBox (strict)"(error in=w3240, "Active Row"=w3239) -> (error out=w3238:errorcluster)  [unwired: 1 in, 1 out]
        n1929 = Select(t=w3244, s=w3243, f=u32 0) -> (s? t:f=w3241:u32)
        n1930 = property on="Signals to Plot" class="LstBox (strict)"(error in=w3238, "CellFontColor"=w3241, "SelColor"=w3237, "CellBG"=w3237, "CellFontSize"=u32 20 ("Active Row:Cell Font:Size"), "CellFontBold"=TRUE ("Active Row:Cell Font:Bold")) -> ()  [unwired: 1 in, 2 out]
      }
      event "BD 1 Frequency 1 (MHz)", "BD 1 Frequency 2 (MHz)", "BD 1 Frequency 3 (MHz)", "BD 2 Frequency 1 (MHz)", "BD 2 Frequency 2 (MHz)", "BD 2 Frequency 3 (MHz)", "Trap Delta (MHz)": Value Change {
        n1931 = event-data() -> ("CtlRef"=w3253:refnum<vi>)  [unwired: 6 out]
        n1932 = control-ref of="Trap Delta (MHz)"() -> (w3252:refnum<vi>)
        n1933 = Equal?(x=w3252, y=w3253) -> (x = y?=w3251:bool)
        n1934 = case shown="False" "Oscillate Set 1" {
          tunnel: w3256 -> [w3276 _]
          tunnel: [w3275 w3279] -> w3255
          tunnel: w3254 -> [w3274 w3279]
          tunnel: w3251 -> [w3259 _]
          frame False {
            n1935 = local read "BD 1 Frequency 2 (MHz)"() -> (w3263:dbl)
            n1936 = local read "BD 1 Frequency 1 (MHz)"() -> (w3261:dbl)
            n1937 = Subtract(x=w3263, y="Trap Delta (MHz)") -> (x-y=w3260:dbl)
            n1938 = Select(t=w3260, s=w3259, f=w3261) -> (s? t:f=w3258:dbl)
            n1939 = local read "Y RF Frequency Limits (MHz)"() -> (w3264:T16)
            n1940 = local read "X RF Frequency Limits (MHz)"() -> (w3265:T16)
            n1941 = local read "BD 1 Frequency 3 (MHz)"() -> (w3277:dbl)
            n1942 = local write "BD 1 Frequency 1 (MHz)"(w3258) -> ()
            n1943 = local read "BD 2 Frequency 1 (MHz)"() -> (w3268:dbl)
            n1944 = local read "BD 2 Frequency 2 (MHz)"() -> (w3267:dbl)
            n1945 = local read "BD 2 Frequency 3 (MHz)"() -> (w3278:dbl)
            n1946 = call "set RF board frequency - interlace.vi"("Board 2 Frequency Limits"=w3264, "Board 1 Frequency Limits"=w3265, "error in"=w3274, "FPGA VI Reference In"=w3276, "Board 2 Frequency 3 (MHz)"=w3278, "Board 1 Frequency 3 (MHz)"=w3277, "Board 2 Frequency 2 (MHz)"=w3267, "Board 2 Frequency 1 (MHz)"=w3268, "Board 1 Frequency 2 (MHz)"=w3263, "Board 1 Frequency 1  (MHz)"=w3258) -> ("error out"=w3275:errorcluster)  [unwired: 1 out]
            n1947 = Subtract(x=w3268, y=w3267) -> (x-y=w3272:dbl)
            n1948 = Subtract(x=w3258, y=w3263) -> (x-y=w3273:dbl)
            n1949 = Square(x=w3272) -> (x^2=w3270:dbl)
            n1950 = Square(x=w3273) -> (x^2=w3271:dbl)
            n1951 = Add(x=w3271, y=w3270) -> (x+y=w3269:dbl)
            n1952 = Square Root(x=w3269) -> (sqrt(x)=w3266:dbl)
            n1953 = local write "Trap Delta (MHz)"(w3266) -> ()
            n1954 = property on="Initial delta (MHz)" class="DigNum (strict)"("Val(Sgnl)"=w3266) -> ()  [unwired: 2 in, 2 out]
          }
          frame True {
          }
        }
      }
      event "Round T1 X": Value Change {
        n1955 = event-data() -> ()  [unwired: 7 out]
        n1956 = local read "BD 1 Frequency 1 (MHz)"() -> (w3282:dbl)
        n1957 = Round To Nearest(number=w3282) -> (nearest integer value=w3281:dbl)
        n1958 = property on="BD 1 Frequency 1 (MHz)" class="DigNum (strict)"("Val(Sgnl)"=w3281) -> ()  [unwired: 2 in, 2 out]
      }
      event "Round T2 X": Value Change {
        n1959 = event-data() -> ()  [unwired: 7 out]
        n1960 = local read "BD 1 Frequency 2 (MHz)"() -> (w3284:dbl)
        n1961 = Round To Nearest(number=w3284) -> (nearest integer value=w3283:dbl)
        n1962 = property on="BD 1 Frequency 2 (MHz)" class="DigNum (strict)"("Val(Sgnl)"=w3283) -> ()  [unwired: 2 in, 2 out]
      }
      event "Stop All": Value Change {
        n1963 = event-data() -> ()  [unwired: 7 out]
        n1964 = local read "Stop All"() -> (w3286:bool)
      }
      event "Delayed Interlace Start": Value Change {
        n1965 = event-data() -> ()  [unwired: 7 out]
        n1966 = flat-sequence {
          frame #0 {
            n1967 = Multiply(x="Delay to Interlace (s)", y=1000.0) -> (x*y=w3289:dbl)
            n1968 = Wait (ms)(milliseconds to wait=w3289) -> ()  [unwired: 1 out]
          }
          frame #1 {
            n1969 = property on="Green laser mode" class="RadioBtnsControl (strict)"("Val(Sgnl)"=enum32{"Laser ON", "Laser OFF", "Interlace"}."Interlace" ("Value (Signaling)")) -> ()  [unwired: 2 in, 2 out]
          }
        }
      }
      event "BD 1 Amplitude 1 (%)", "BD 1 Amplitude 2 (%)", "BD 1 Amplitude 3 (%)", "BD 2 Amplitude 1 (%)", "BD 2 Amplitude 2 (%)", "BD 2 Amplitude 3 (%)", "Trap 1 ON", "Trap 2 ON", "Trap 3 ON", "Feedback On/Off", "All FB On/Off": Value Change {
        w3313 = i16 1 ("f")
        n1970 = event-data() -> ()  [unwired: 7 out]
        n1971 = local write "Trap 1 (ON/OFF)"("Trap 1 ON") -> ()
        n1972 = local write "Trap 2 (ON/OFF)"("Trap 2 ON") -> ()
        n1973 = Boolean To (0,1)(Boolean="Trap 3 ON") -> (0, 1=w3314:i16)
        n1974 = Boolean To (0,1)(Boolean="Trap 1 ON") -> (0, 1=w3315:i16)
        n1975 = Boolean To (0,1)(Boolean="Trap 2 ON") -> (0, 1=w3316:i16)
        n1976 = Select(t=w3316, s="Trap ON/OFF X or Y Amp?", f=w3313) -> (s? t:f=w3311:i16)
        n1977 = Select(t=w3315, s="Trap ON/OFF X or Y Amp?", f=w3313) -> (s? t:f=w3312:i16)
        n1978 = Select(t=w3314, s="Trap ON/OFF X or Y Amp?", f=w3313) -> (s? t:f=w3310:i16)
        n1979 = Select(t=w3313, s="Trap ON/OFF X or Y Amp?", f=w3316) -> (s? t:f=w3308:i16)
        n1980 = Select(t=w3313, s="Trap ON/OFF X or Y Amp?", f=w3315) -> (s? t:f=w3309:i16)
        n1981 = Select(t=w3313, s="Trap ON/OFF X or Y Amp?", f=w3314) -> (s? t:f=w3307:i16)
        n1982 = And(x="All FB On/Off", y="Feedback On/Off") -> (x .and. y?=w3305:cluster{"Set 1":bool, "Set 2":bool})
        n1983 = local read "BD 1 Amplitude 1 (%)"() -> (w3325:dbl)
        n1984 = local read "BD 1 Amplitude 2 (%)"() -> (w3324:dbl)
        n1985 = local read "BD 1 Amplitude 3 (%)"() -> (w3323:dbl)
        n1986 = Unbundle By Name(w3305) -> ("Set 1"=w3300:bool, "Set 2"=w3297:bool)
        n1987 = local read "Y RF Amplitude Limits (%)"() -> (w3293:T16)
        n1988 = local read "X RF Amplitude Limits (%)"() -> (w3294:T16)
        n1989 = local read "BD 2 Amplitude 1 (%)"() -> (w3326:dbl)
        n1990 = local read "BD 2 Amplitude 2 (%)"() -> (w3327:dbl)
        n1991 = local read "BD 2 Amplitude 3 (%)"() -> (w3328:dbl)
        n1992 = And(x="Trap 2 ON", y=w3297) -> (x .and. y?=w3295:bool)
        n1993 = And(x="Trap 1 ON", y=w3300) -> (x .and. y?=w3298:bool)
        n1994 = Multiply(x=w3312, y=w3325) -> (x*y=w3320:dbl)
        n1995 = Multiply(x=w3324, y=w3311) -> (x*y=w3318:dbl)
        n1996 = Multiply(x=w3323, y=w3310) -> (x*y=w3319:dbl)
        n1997 = Multiply(x=w3326, y=w3309) -> (x*y=w3329:dbl)
        n1998 = Multiply(x=w3327, y=w3308) -> (x*y=w3330:dbl)
        n1999 = Multiply(x=w3328, y=w3307) -> (x*y=w3331:dbl)
        n2000 = call "set RF board amplitude - interlace.vi"("Board 2 Amplitude Limits"=w3293, "Board 1 Amplitude Limits"=w3294, "error in"=w3321, "FPGA VI Reference In"=w3322, "Board 2 Amplitude 3 (%)"=w3331, "Board 1 Amplitude 3 (%)"=w3319, "Board 2 Amplitude 2 (%)"=w3330, "Board 2 Amplitude 1 (%)"=w3329, "Board 1 Amplitude 2 (%)"=w3318, "Board 1 Amplitude 1 (%)"=w3320) -> ("error out"=w3302:errorcluster, "FPGA VI Reference Out"=w3303:T19)
        n2001 = xnode "Read/Write Control"("FPGA VI Reference In"=w3303, "error in"=w3302, "FB On/Off Set 1"=w3298, "FB On/Off Set 2"=w3295) -> ("error out"=w3301:errorcluster)  [unwired: 1 out]
      }
      event "Load parameters": Value Change {
        n2002 = event-data() -> ()  [unwired: 7 out]
        n2003 = property on="Saved AOD Raster Scan Parameter Sets" class="Arr (strict)"() -> ("Index Values"=w3342:u32[])  [unwired: 2 in, 2 out]
        n2004 = Index Array(array=w3342, index=0) -> (element=w3339:u32)
        n2005 = local write "Load parameters"(FALSE ("Load parameters")) -> ()
        n2006 = Index Array(array="Saved AOD Raster Scan Parameter Sets", index=w3339) -> (element=w3338:T45)
        n2007 = Unbundle By Name(w3338) -> ("Scan Range AOD (nm) 2"=w3337:dbl, "Step Size AOD (nm) 2"=w3336:dbl, "Scan Speed AOD (nm/s) 2"=w3335:dbl, "Number of scans (AOD) 2"=w3334:u16)
        n2008 = flat-sequence {
          tunnel: w3337 -> [w3345]
          tunnel: w3336 -> [w3344]
          tunnel: w3335 -> [w3343]
          tunnel: w3334 -> [w3346]
          frame #0 {
            n2009 = local write "Scan Speed (nm/s)"(w3343) -> ()
            n2010 = local write "Scan Range (nm)"(w3345) -> ()
            n2011 = local write "Step Size (nm)"(w3344) -> ()
          }
          frame #1 {
            n2012 = property on="Number of F/B Scans (AOD)" class="DigNum (strict)"("Val(Sgnl)"=w3346) -> ()  [unwired: 2 in, 2 out]
          }
        }
      }
      event "Trap 1 (ON/OFF)", "Trap 2 (ON/OFF)": Value Change {
        n2013 = event-data() -> ()  [unwired: 7 out]
        n2014 = property on="Trap 2 ON" class="Bool (strict)"("Val(Sgnl)"="Trap 2 (ON/OFF)") -> ()  [unwired: 2 in, 2 out]
        n2015 = property on="Trap 1 ON" class="Bool (strict)"("Val(Sgnl)"="Trap 1 (ON/OFF)") -> ()  [unwired: 2 in, 2 out]
      }
      event "DIO count 1 (ticks)", "DIO count 2 (ticks)", "DIO count 3 (ticks)", "Interlace", "Number Interlace Sets", "Not-Interlacing Set": Value Change {
        n2016 = event-data() -> ()  [unwired: 7 out]
        n2017 = local read "DIO count 3 (ticks)"() -> (w3359:u32)
        n2018 = local read "DIO count 1 (ticks)"() -> (w3361:u32)
        n2019 = local read "DIO count 2 (ticks)"() -> (w3360:u32)
        n2020 = To Unsigned Byte Integer(number="Not-Interlacing Set") -> (unsigned 8bit integer=w3350:u8)
        n2021 = Add(x=w3350, y=u8 1) -> (x+y=w3354:u8)
        n2022 = xnode "Read/Write Control"("FPGA VI Reference In"=w3365, "error in"=w3363, "DIO count 1 (ticks)"=w3361, "DIO count 2 (ticks)"=w3360, "DIO count 3 (ticks)"=w3359, "Interlace ON/OFF"="Interlace", "Number Interlace Cycles"="Number Interlace Sets", "Interlace Off Parameters"=w3354) -> ("error out"=w3364:errorcluster)  [unwired: 1 out]
        n2023 = Build Array(w3361, w3360, w3359) -> (w3352:u32[])
        n2024 = Split 1D Array(array=w3352, index="Number Interlace Sets") -> (first subarray=w3362:u32[])  [unwired: 1 out]
        n2025 = Index Array(array=w3352, index=w3350) -> (element=w3351:u32)
        n2026 = Add Array Elements(numeric array=w3362) -> (sum=w3356:u32)
        n2027 = Select(t=w3356, s="Interlace", f=w3351) -> (s? t:f=→"Total Counts (ticks)":u32)
      }
      event "Reset Feedback": Value Change {
        n2028 = event-data() -> ()  [unwired: 7 out]
        n2029 = Unbundle By Name("Reset Feedback") -> ("Set 1"=w3369:bool, "Set 2"=w3368:bool)
        n2030 = xnode "Read/Write Control"("FPGA VI Reference In"=w3371, "error in"=w3366, "FB Reset Set 1"=w3369, "FB Reset Set 2"=w3368) -> ("error out"=w3367:errorcluster)  [unwired: 1 out]
      }
      event "PID Gains": Value Change {
        n2031 = event-data() -> ()  [unwired: 7 out]
        n2032 = Unbundle By Name("PID Gains") -> ("Set 1"=w3375:T14, "Set 2"=w3374:T14)
        n2033 = xnode "Read/Write Control"("FPGA VI Reference In"=w3376, "error in"=w3372, "FB Gains Set 1"=w3375, "FB Gains Set 2"=w3374) -> ("error out"=w3373:errorcluster)  [unwired: 1 out]
      }
      event "AI2 to Setpoint", "Setpoints (V)": Value Change {
        n2034 = event-data() -> ()  [unwired: 7 out]
        n2035 = xnode "Read/Write Control"("FPGA VI Reference In"=w3382, "error in"=w3378) -> ("FPGA VI Reference Out"=w3381:T19, "error out"=w3380:errorcluster, "AI2 Y Sum Set 1"=w3389:i16, "AI2 Y Sum Set 2"=w3388:i16)
        n2036 = Cluster To Array(cluster="AI2 to Setpoint") -> (array=w3392:bool[])
        n2037 = local read "AI2 (V)"() -> (w3390:cluster{"Set 1":dbl, "Set 2":dbl})
        n2038 = Or Array Elements(Boolean array=w3392) -> (logical OR=w3393:bool)
        n2039 = Bundle By Name(cluster=w3390, "Set 1"=w3389, "Set 2"=w3388) -> (w3387:cluster{"Set 1":dbl, "Set 2":dbl})
        n2040 = Divide(x=w3387, y=3276.7) -> (x/y=w3386:cluster{"Set 1":dbl, "Set 2":dbl})
        "AI2 (V)" <- w3386
        n2041 = case shown="True" w3393 {
          tunnel: [w3396 w3413] -> w3385
          tunnel: "AI2 to Setpoint" -> [_ w3409]
          tunnel: "Setpoints (V)" -> [w3397 w3412]
          tunnel: w3386 -> [_ w3406]
          frame False {
            n2042 = Multiply(x=3276.7, y=w3397) -> (x*y=w3398:cluster{"Set 1":dbl, "Set 2":dbl})
            n2043 = To Word Integer(number=w3398) -> (16bit integer=w3396:cluster{"Set 1":i16, "Set 2":i16})
          }
          frame True {
